vi "worksheet protect.vi"(8 "error in (no error)":errorcluster, 9 "options":T1, 10 "password":string, 11 "worksheet":u32) -> (0 "error out":errorcluster, 1 "options out":T1)   [LabVIEW 8.6]
doc: "void worksheet_protect(lxw_worksheet worksheet, const char *password, lxw_protection *options);"
uses:
  pending_lvxlsxwriter/xlsxwriter.dll
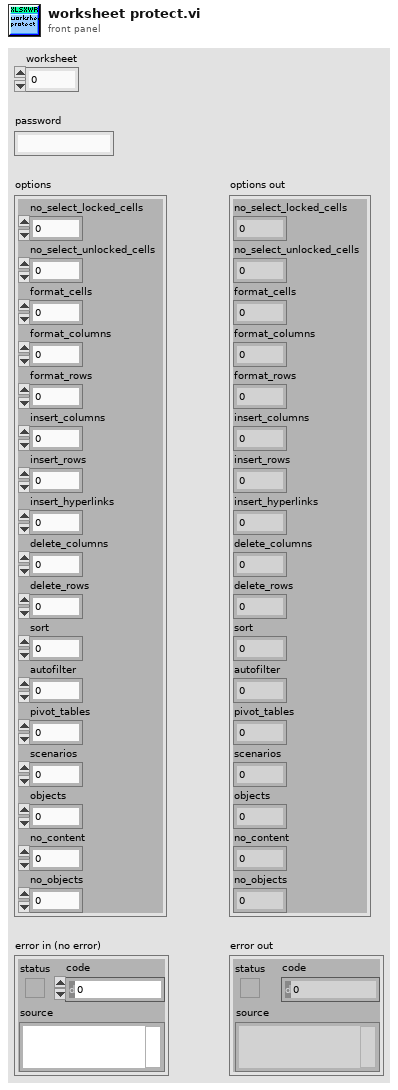
[diagram p1: front panel]
types:
  T1 = cluster{"no_select_locked_cells":u8, "no_select_unlocked_cells":u8, "format_cells":u8, "format_columns":u8, "format_rows":u8, "insert_columns":u8, "insert_rows":u8, "insert_hyperlinks":u8, "delete_columns":u8, "delete_rows":u8, "sort":u8, "autofilter":u8, "pivot_tables":u8, "scenarios":u8, "objects":u8, "no_content":u8, "no_objects":u8}
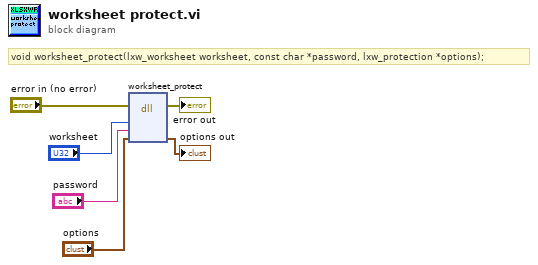
[diagram p0: block diagram]
diagram:
  # "void worksheet_protect(lxw_worksheet worksheet, const char *password, lxw_protection *options);"
  n1 = dll-call lib="C:/Users/WDAGUtilityAccount/Desktop/pending_lvxlsxwriter/xlsxwriter.*" fn="worksheet_protect"(error in="error in (no error)", "worksheet"="worksheet", "password"="password", "options"="options") -> (error out=→"error out":errorcluster, "options"=→"options out":T1)  [unwired: 5 in, 1 out]
